vi "getdrive joystick.vi"(11 "Robot filed orientation (deg)":dbl) -> (2 "drive joystick buttons":bool[](array[boolean]), 3 "drive joystick values":dbl[](array[numeric]))   [LabVIEW 2018]
uses:
  <vilib>/Rock Robotics/Network Tables/NT Write Numeric Array.vi
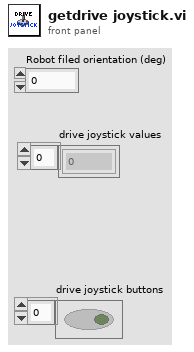
[diagram p1: front panel]
types:
  T1 = typedef "DriveJoystickButtonMapping.ctl" = cluster{"relative encoders?":bool, "zero relative encoder":bool, "reset field orientation":bool, "use field orientation":bool}
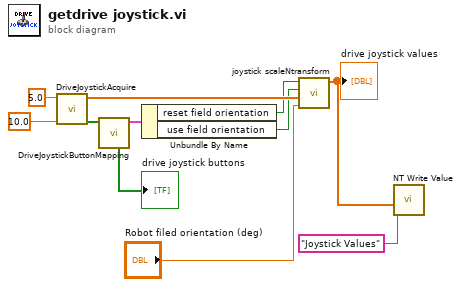
[diagram p0: block diagram]
diagram:
  n1 = call "DriveJoystickAcquire.vi"("Rotation Joystick Deadband %"=10.0, "XY Joystick Deadband %"=5.0) -> ("Drive Joystick Buttons"=w7:bool[], "Drive Joystick Values"=w8:dbl[])  [unwired: 8 in]
  n2 = call "DriveJoystickButtonMapping.vi"("drive joystick buttons"=w7) -> ("DriveJoystickButtonMapping"=w5:T1, "drive joystick buttons indicator"=→"drive joystick buttons":bool[])  [unwired: 9 in]
  n3 = Unbundle By Name(w5) -> ("reset field orientation"=w4:bool, "use field orientation"=w3:bool)
  n4 = call "joystick scaleNtransform.vi"("robot field orientation (deg)"="Robot filed orientation (deg)", "joystick values"=w8, "use filed orientation"=w3, "reset field orientation"=w4) -> ("Transformed joystick values"=w2:dbl[])  [unwired: 7 in]
  "drive joystick values" <- w2
  n5 = call-poly <vilib>:"NT Write Value.vi"("Numeric Array"=w2, "Name"="Joystick Values") -> ()  [unwired: 9 in, 1 out]
